vi "Client Test.vi"() -> ()   [LabVIEW 2019, in "TempController_client.lvlib" / "TempController_client.lvclass"]
uses:
  TempController_client.lvclass
  RPC Messages/MeasureResponse/MeasureResponse_Data.ctl
  RPC Messages/ControllerSettingsRequest/ControllerSettingsRequest_Data.ctl
  RPC Messages/MeasureRequest/MeasureRequest_Data.ctl
panel:
  in  "address":string="localhost:50051"
  in  "Request Data":T1={"temperature_setpoint"=25.0, "unit"=0, "enabled"=TRUE}
  out "Temperature":T2
  out "error out":errorcluster
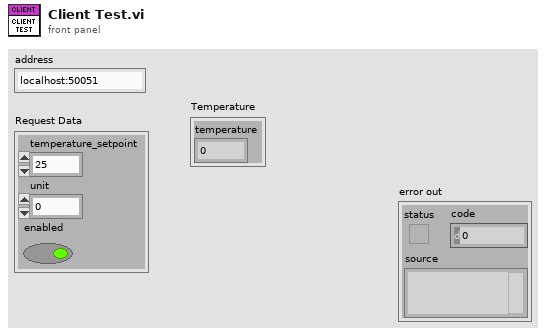
[diagram p1: front panel]
types:
  T1 = typedef "TempController_client.lvlib/TempController_client.lvclass/ControllerSettingsRequest_Data.ctl" = cluster{"temperature_setpoint":dbl, "unit":i32, "enabled":bool}
  T2 = typedef "TempController_client.lvlib/TempController_client.lvclass/MeasureResponse_Data.ctl" = cluster{"temperature":dbl}
  T3 = typedef "TempController_client.lvlib/TempController_client.lvclass/MeasureRequest_Data.ctl" = cluster{"unit":i32}
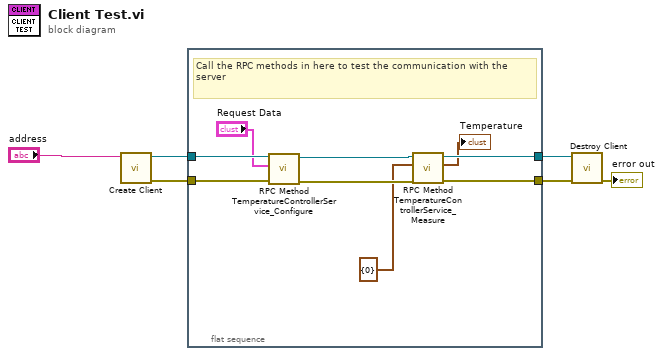
[diagram p0: block diagram]
diagram:
  n1 = call "Create Client.vi"("address"="address") -> ("error out"=w2:errorcluster, "gRPC Client out"=w4:refnum<class "TempController_client.lvclass">)  [unwired: 9 in]
  n2 = flat-sequence {
    tunnel: [w13] -> w5
    tunnel: w4 -> [w15]
    tunnel: [w10] -> w3
    tunnel: w2 -> [w12]
    frame #0 {
      # "Call the RPC methods in here to test the communication with the server"
      n3 = call "RPC Method TemperatureControllerService_Configure.vi"("error in (no error)"=w12, "Request Data"="Request Data", "gRPC Client in"=w15) -> ("error out"=w11:errorcluster, "gRPC Client out"=w14:refnum<class "TempController_client.lvclass">)  [unwired: 6 in, 1 out]
      n4 = call "RPC Method TemperatureControllerService_Measure.vi"("error in (no error)"=w11, "Request Data"=T3 {"unit"=0}, "gRPC Client in"=w14) -> ("error out"=w10:errorcluster, "Response Data"=→"Temperature":T2, "gRPC Client out"=w13:refnum<class "TempController_client.lvclass">)  [unwired: 6 in]
    }
  }
  n5 = call "Destroy Client.vi"("error in (no error)"=w3, "gRPC Client in"=w5) -> ("error out"=→"error out":errorcluster)  [unwired: 8 in, 1 out]
